vi "Read Color Area Size.vi"(8 "error in (no error)":errorcluster, 11 "ColorRamp.lvclass in":refnum<class "ColorRamp.lvclass">) -> (0 "error out":errorcluster, 2 "ColorAreaSize":T1, 3 "ColorRamp.lvclass out":refnum<class "ColorRamp.lvclass">)   [LabVIEW 2015, in "ColorRamp.lvclass"]
uses:
  ColorRamp.lvclass
  <vilib>/Utility/miscctls.llb/LVBoundsTypeDef.ctl
  ColorRamp.lvclass/ColorRamp.ctl
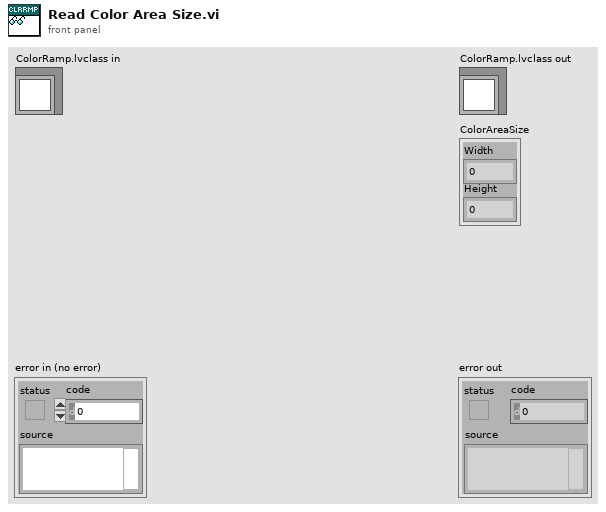
[diagram p1: front panel]
types:
  T1 = typedef "LVBoundsTypeDef.ctl" = cluster{"Width":u32, "Height":u32}
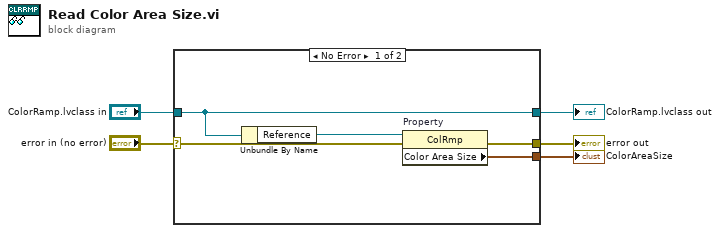
[diagram p0: block diagram]
diagram:
  n1 = case shown="No Error" "error in (no error)" {
    selector: "error in (no error)" -> [w6 w12]
    tunnel: [w9 w12] -> w4
    tunnel: [w8 w11] -> w2
    tunnel: "ColorRamp.lvclass in" -> [w8 w11]
    tunnel: [w10 _] -> w1
    frame No Error {
      n2 = Unbundle By Name(w8) -> ("Reference"=w7:refnum<vi>)
      n3 = property on="Property" class="ColRmp"(reference=w7, error in=w6) -> (error out=w9:errorcluster, "Color Area Size"=w10:T1)  [unwired: 1 out]
    }
    frame Error {
    }
  }
  "error out" <- w4
  "ColorRamp.lvclass out" <- w2
  "ColorAreaSize" <- w1
